vi "OpenOrCreateTestDB.vi"(8 "error in (no error)":errorcluster, 10 "path to db":path, 11 "SQLite in":refnum<class "Kopie von SQLite.lvclass">) -> (0 "error out":errorcluster, 1 "DB Path":path, 2 "DB Path":string, 3 "SQLite out":refnum<class "Kopie von SQLite.lvclass">)   [LabVIEW 2017, in "Kopie von SQLite.lvclass"]
uses:
  Kopie von SQLite.lvclass
  Kopie von SQLite.lvclass/Kopie von SQLite.ctl
  <vilib>/drjdpowell/SQLite Library/SQL Connection/Open (path).vi
  <vilib>/drjdpowell/SQLite Library/SQL Connection/Open (string).vi
  <vilib>/AdvancedString/Path To Command Line String.vi
  <vilib>/drjdpowell/SQLite Library/SQL Connection/Connection.lvclass
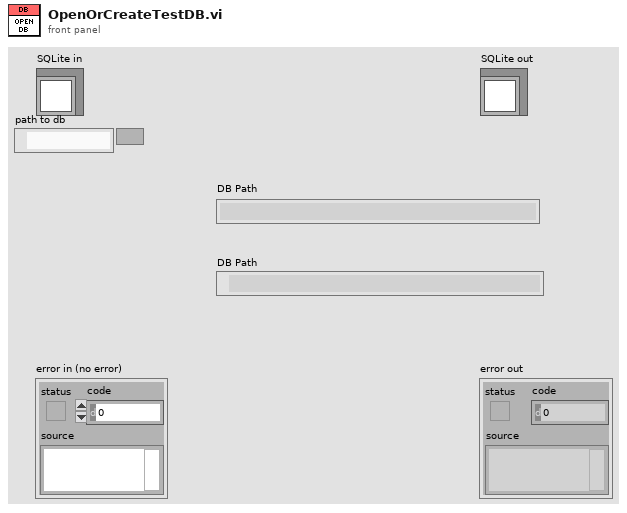
[diagram p1: front panel]
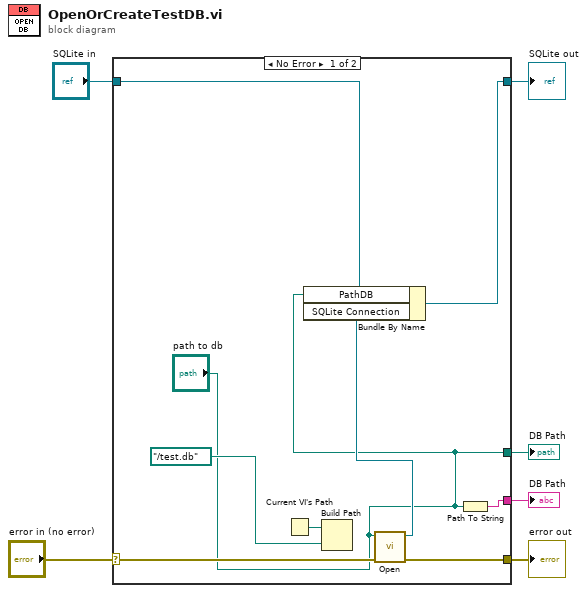
[diagram p0: block diagram]
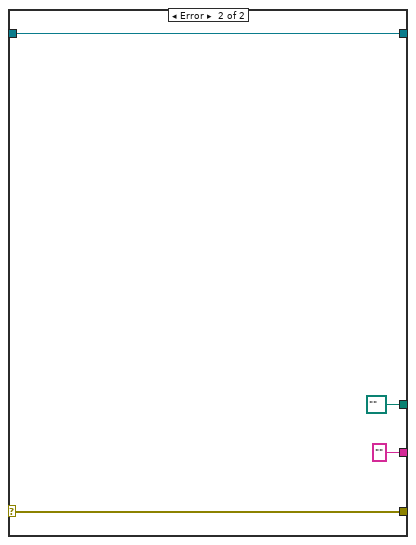
[diagram p2: hidden frame]
diagram:
  n1 = case shown="No Error" "error in (no error)" {
    selector: "error in (no error)" -> [w12 w19]
    tunnel: [w11 w19] -> w5
    tunnel: [w8 w18] -> w3
    tunnel: "SQLite in" -> [w10 w18]
    tunnel: [w13 ""] -> w2
    tunnel: ["path to db" path ""] -> w1
    frame No Error {
      n2 = Current VI's Path() -> (path=w15:path)
      n3 = Build Path(base path=w15, name or relative path=path "../test.db") -> ()  [unwired: 1 out]
      n4 = call-poly <vilib>:"Open.vi"("error in (no error)"=w12, "db file"="path to db") -> ("error out"=w11:errorcluster, "SQLite Connection out"=w9:refnum<class "Connection.lvclass">)  [unwired: 8 in]
      n5 = Bundle By Name(cluster=w10, "PathDB"="path to db", "SQLite Connection"=w9) -> (w8:refnum<class "Kopie von SQLite.lvclass">)
      n6 = Path To String(path="path to db") -> (string=w13:string)
    }
    frame Error {
    }
  }
  "error out" <- w5
  "SQLite out" <- w3
  "DB Path" <- w2
  "DB Path" <- w1
